vi "IO test.vi"() -> ()   [LabVIEW 2016]
uses:
  Classes/Controller/I-O/NI-DAQ Folder/NI-DAQ.lvclass
panel:
  in  "IO turn off":bool
  out "subarray":bool[](array[boolean])
  in  "IO control":bool
  in  "stop":bool
  in  "values":bool[](array[boolean])
  in  "indices":i32[](array[numeric])
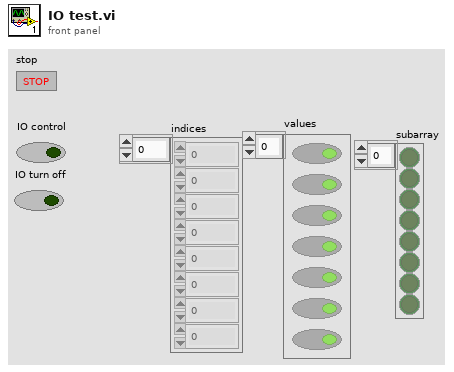
[diagram p1: front panel]
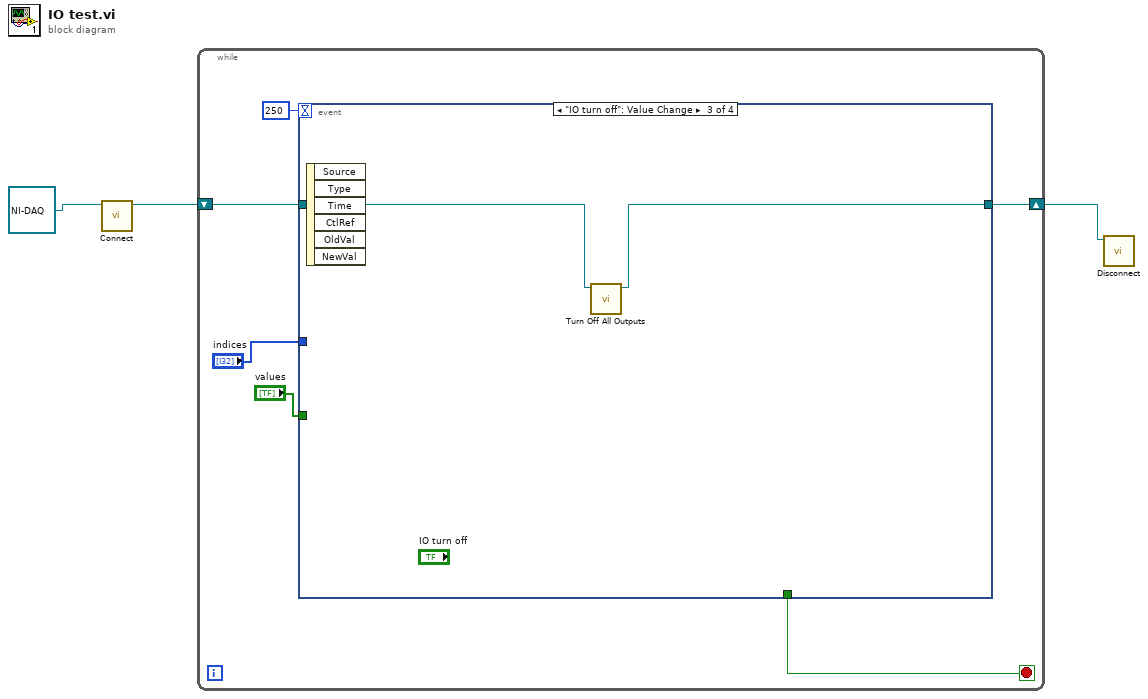
[diagram p0: block diagram]
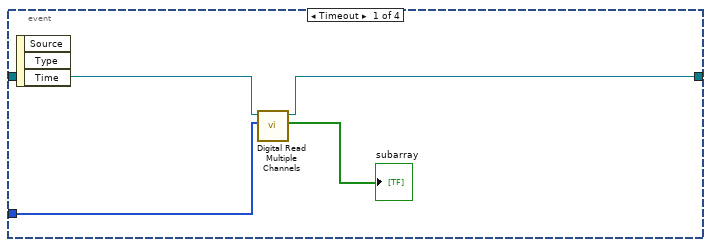
[diagram p2: hidden frame]
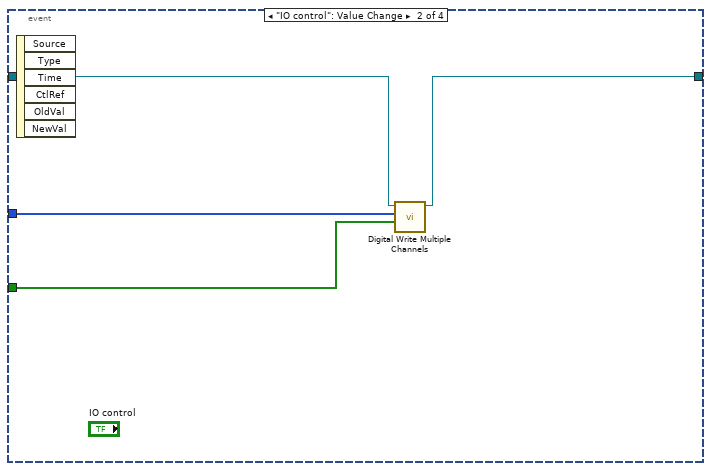
[diagram p3: hidden frame]
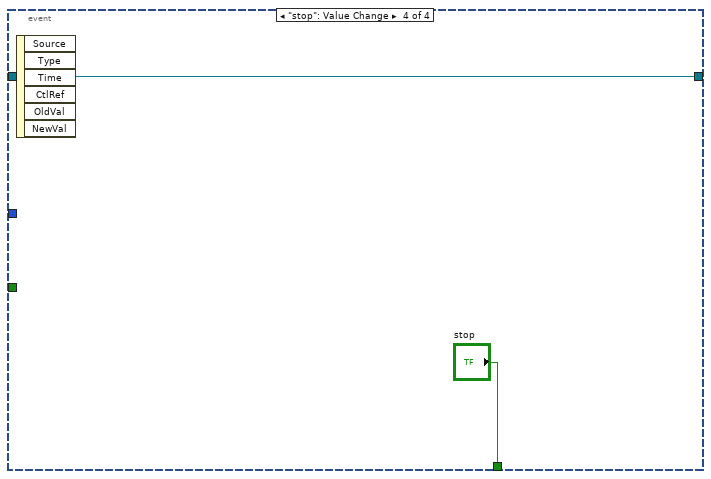
[diagram p4: hidden frame]
diagram:
  n1 = call-dynamic "Connect.vi"("NI-DAQ in"=refnum<class "NI-DAQ.lvclass"> refnum ("NI-DAQ.lvclass")) -> ("NI-DAQ out"=w1:refnum<class "NI-DAQ.lvclass">)  [unwired: 9 in, 1 out]
  n2 = while {
    shift-right: [w7] -> w2
    shift-left: w1 -> [w8]
    stop <- w9 stop-if-true
    n3 = event shown="[2] \"IO turn off\": Value Change" {
      selector: _ -> [_ _ _ _]
      dyn-events: _ -> [_ _ _ _]
      timeout: 250 -> [_ _ _ _]
      tunnel: [_ _ _ "stop"] -> w9
      tunnel: w8 -> [w12 w15 w19 w20]
      tunnel: [w13 w14 w18 w20] -> w7
      tunnel: "values" -> [_ w17 _ _]
      tunnel: "indices" -> [w11 w16 _ _]
      event Timeout {
        n4 = event-data() -> ()  [unwired: 1 in, 3 out]
        n5 = call-dynamic "Digital Read Multiple Channels.vi"("Array"=w11, "NI-DAQ in"=w12) -> ("subarray"=→"subarray":bool[], "NI-DAQ out"=w13:refnum<class "NI-DAQ.lvclass">)  [unwired: 7 in, 1 out]
      }
      event "IO control": Value Change {
        n6 = event-data() -> ()  [unwired: 1 in, 6 out]
        n7 = call-dynamic "Digital Write Multiple Channels.vi"("Values"=w17, "Indices"=w16, "NI-DAQ in"=w15) -> ("NI-DAQ out"=w14:refnum<class "NI-DAQ.lvclass">)  [unwired: 7 in, 1 out]
      }
      event "IO turn off": Value Change {
        n8 = event-data() -> ()  [unwired: 1 in, 6 out]
        n9 = call-dynamic "Turn Off All Outputs.vi"("NI-DAQ in"=w19) -> ("NI-DAQ out"=w18:refnum<class "NI-DAQ.lvclass">)  [unwired: 9 in, 1 out]
      }
      event "stop": Value Change {
        n10 = event-data() -> ()  [unwired: 1 in, 6 out]
      }
    }
  }
  n11 = call-dynamic "Disconnect.vi"("I-O in"=w2) -> ()  [unwired: 9 in, 1 out]
